vi "USB Open.vi"(8 "error in (no error)":errorcluster) -> (0 "error out":errorcluster, 3 "function return":i32)   [LabVIEW 2011, in "Stats32.lvlib"]
doc: "LIBRARY_API int USB_Open();"
uses:
  Stats32.lvlib
  Stats/Release/Win32/Stats32.dll
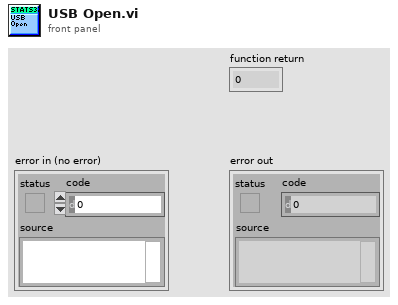
[diagram p1: front panel]
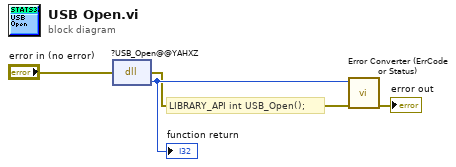
[diagram p0: block diagram]
diagram:
  # "LIBRARY_API int USB_Open();"
  n1 = dll-call lib="C:/Programming/Stats/Stats/Release/Win32/Stats32.*" fn="?USB_Open@@YAHXZ"(error in="error in (no error)") -> (error out=w2:errorcluster, w4:i32)  [unwired: 2 in, 1 out]
  "function return" <- w4
  n2 = call "Error Converter (ErrCode or Status).vi"("error in (no error)"=w2, "error code"=w4) -> ("error out"=→"error out":errorcluster)  [unwired: 9 in]
